vi "Sort Folders by Depth.vi"(11 "Folders In":T1[](array[typedef])) -> (3 "Sorted Folders":T1[](array[typedef]))   [LabVIEW 2020, in "Negentropic IDE.lvlib"]
uses:
  Negentropic IDE.lvlib
  Folder Config.ctl
  Scope.ctl
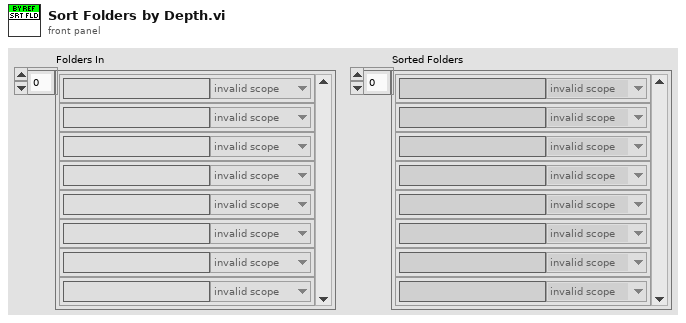
[diagram p1: front panel]
types:
  T1 = typedef "Negentropic IDE.lvlib/Folder Config.ctl" = cluster{"Path":string, "Scope":T2}
  T2 = typedef "Negentropic IDE.lvlib/Scope.ctl" = enum32{"invalid scope", "public", "private", "protected", "community"}
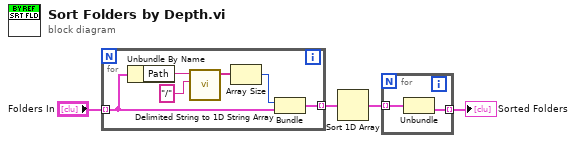
[diagram p0: block diagram]
diagram:
  n1 = for {
    tunnel: "Folders In" -> [w7] mode=indexing
    tunnel: [w5] -> w3 mode=indexing
    n2 = Unbundle By Name(w7) -> ("Path"=w10:string)
    n3 = call <vilib>:"Delimited String to 1D String Array.vi"("delimiter"="/", "delimited string"=w10) -> ("string array"=w8:string[])  [unwired: 9 in]
    n4 = Array Size(array=w8) -> (size(s)=w6:i32)
    n5 = Bundle(w6, "Folder Config"=w7) -> (w5:cluster{i32, "Folder Config":T1})  [unwired: 1 in]
  }
  n6 = Sort 1D Array(array=w3) -> (sorted array=w2:cluster{i32, "Folder Config":T1}[])
  n7 = for {
    tunnel: w2 -> [w12] mode=indexing
    tunnel: [w11] -> w1 mode=indexing
    n8 = Unbundle(w12) -> ("Folder Config"=w11:T1)  [unwired: 1 out]
  }
  "Sorted Folders" <- w1
